vi "Before.vi"(7 "Actor in":refnum<class "Actor.lvclass">, 8 "Error in":errorcluster, 10 "Msg DVR in":refnum<data-value>) -> (0 "Error out":errorcluster, 2 "Msg DVR out":refnum<data-value>, 5 "Actor out":refnum<class "Actor.lvclass">)   [LabVIEW 2020, in "_Template.lvlib" / "Templates.lvlib" / "TEMPLATE jettl Msg.lvlib" / "TEMPLATE Msg Contents.lvclass"]
uses:
  TEMPLATE Msg Contents.lvclass
  TEMPLATE Msg Contents.lvclass/TEMPLATE Msg Contents.ctl
  TEMPLATE jettl Msg/TEMPLATE jettl Msg.lvclass
  jettl/jettl/Actor/Actor.lvclass
  jettl/jettl/Unified Actor Relation.ctl
  jettl/jettl/jettl.lvlib
  jettl/jettl/Teller.ctl
  jettl/jettl/Msg Contents/Msg Contents.lvclass
  jettl/jettl/Msg.ctl
  jettl/jettl/Msg/Msg.lvclass
panel:
  # "This front panel should not be manipulated."
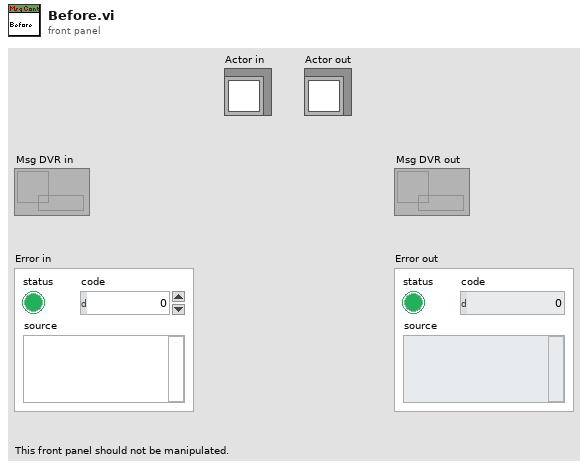
[diagram p1: front panel]
types:
  T1 = typedef "jettl.lvlib/Msg.ctl" = cluster{"Msg":refnum<class "Msg.lvclass">, "Msg Contents":refnum<class "Msg Contents.lvclass">, "Teller":T2}
  T2 = typedef "jettl.lvlib/Teller.ctl" = cluster{"Unified Actor Alias":string, "Unified Actor Relation":T3, "Absolute Time":timestamp, "Relative Time":dbl}
  T3 = typedef "jettl.lvlib/Unified Actor Relation.ctl" = enum16{"Self", "Parent", "Child"}
  T4 = typedef "_Template.lvlib/Templates.lvlib/TEMPLATE jettl Msg.lvlib/Data.ctl" = cluster{"Placeholder Data":bool}
  T5 = typedef "_Template.lvlib/Templates.lvlib/TEMPLATE jettl Msg.lvlib/Metadata.ctl" = cluster{"Placeholder Metadata":bool}
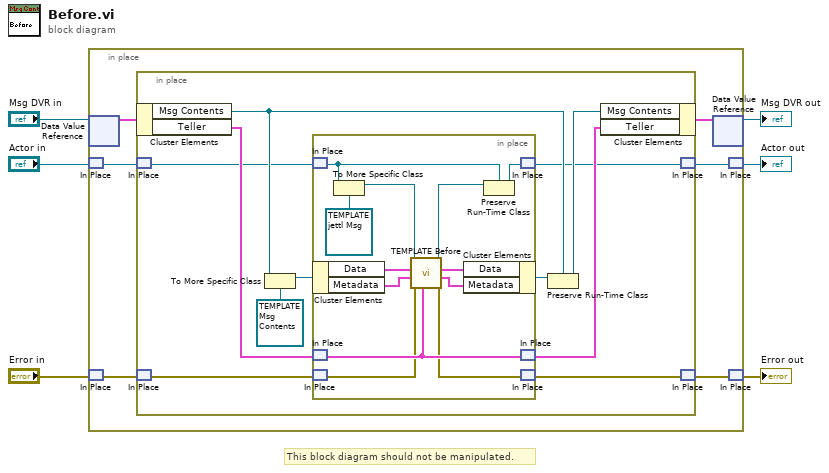
[diagram p0: block diagram]
diagram:
  # "This block diagram should not be manipulated."
  n1 = in-place {
    n2 = in-place-dvr #1("Msg DVR in") -> (w12:T1)  [unwired: 1 out]
    n3 = in-place-match #2("Actor in") -> (w8:refnum<class "Actor.lvclass">)
    n4 = in-place-match #3("Error in") -> (w10:errorcluster)
    n5 = in-place {
      n6 = in-place-cluster #4(w12) -> ("Msg Contents"=w21:refnum<class "Msg Contents.lvclass">, "Teller"=w17:T2)
      n7 = in-place-match #5(w8) -> (w14:refnum<class "Actor.lvclass">)
      n8 = in-place-match #6(w10) -> (w16:errorcluster)
      n9 = To More Specific Class(target class=refnum<class "TEMPLATE Msg Contents.lvclass"> refnum ("_Template.lvlib:Templates.lvlib:TEMPLATE jettl Msg.lvlib:TEMPLATE Msg Input.lvlib:TEMPLATE Msg Input.lvclass"), reference=w21) -> (specific class reference=w22:refnum<class "TEMPLATE Msg Contents.lvclass">)  [unwired: 1 in, 1 out]
      n10 = in-place {
        n11 = in-place-match #7(w14) -> (w24:refnum<class "Actor.lvclass">)
        n12 = in-place-cluster #8(w22) -> ("Data"=w35:T4, "Metadata"=w30:T5)
        n13 = in-place-match #9(w17) -> (w28:T2)
        n14 = in-place-match #10(w16) -> (w27:errorcluster)
        n15 = To More Specific Class(target class=refnum<class "TEMPLATE jettl Msg.lvclass"> refnum ("_Template.lvlib:Templates.lvlib:TEMPLATE jettl Msg.lvlib:TEMPLATE jettl Msg.lvclass"), reference=w24) -> (specific class reference=w33:refnum<class "TEMPLATE jettl Msg.lvclass">)  [unwired: 1 in, 1 out]
        n16 = call-dynamic "TEMPLATE Before.vi"("Teller"=w28, "Error in"=w27, "Metadata in"=w30, "Data in"=w35, "TEMPLATE jettl Msg in"=w33) -> ("Error out"=w26:errorcluster, "Metadata out"=w29:T5, "Data out"=w31:T4, "TEMPLATE jettl Msg out"=w32:refnum<class "TEMPLATE jettl Msg.lvclass">)  [unwired: 3 in]
        n17 = in-place-cluster #8("Data"=w31, "Metadata"=w29) -> (w20:refnum<class "TEMPLATE Msg Contents.lvclass">)
        n18 = Preserve Run-Time Class(object in=w32, 2:w24) -> (object out=w25:refnum<class "Actor.lvclass">)  [unwired: 1 in, 1 out]
        n19 = in-place-match #7(w25) -> (w13:refnum<class "Actor.lvclass">)
        n20 = in-place-match #9(w28) -> (w18:T2)
        n21 = in-place-match #10(w26) -> (w15:errorcluster)
      }
      n22 = Preserve Run-Time Class(object in=w20, 2:w21) -> (object out=w19:refnum<class "Msg Contents.lvclass">)  [unwired: 1 in, 1 out]
      n23 = in-place-cluster #4("Msg Contents"=w19, "Teller"=w18) -> (w11:T1)
      n24 = in-place-match #5(w13) -> (w7:refnum<class "Actor.lvclass">)
      n25 = in-place-match #6(w15) -> (w9:errorcluster)
    }
    n26 = in-place-dvr #1(w11) -> (→"Msg DVR out":refnum<data-value>)  [unwired: 1 out]
    n27 = in-place-match #2(w7) -> (→"Actor out":refnum<class "Actor.lvclass">)
    n28 = in-place-match #3(w9) -> (→"Error out":errorcluster)
  }
